vi "Execute.vi"(8 "error in (no error)":errorcluster, 10 "Abstract Consumer in":refnum<class "Abstract Consumer.lvclass">, 11 "String Request Message in":refnum<class "String Request Message.lvclass">) -> (0 "error out":errorcluster, 1 "Abstract Response out":refnum<class "Abstract Response Message.lvclass">, 2 "Abstract Consumer out":refnum<class "Abstract Consumer.lvclass">, 3 "String Request Message out":refnum<class "String Request Message.lvclass">, 4 "Stop?":bool)   [LabVIEW 2017, in "String Request Message.lvclass"]
uses:
  String Request Message.lvclass
  Consumer/Abstract Consumer/Abstract Consumer.lvclass
  Message/Abstract Response Message/Abstract Response Message.lvclass
  String Request Message.lvclass/String Request Message.ctl
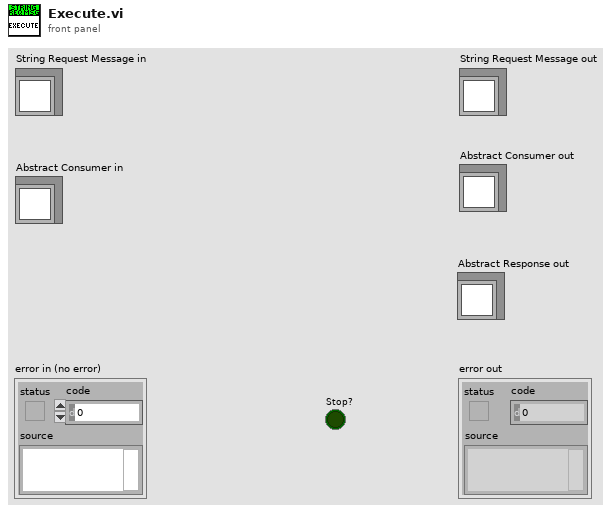
[diagram p1: front panel]
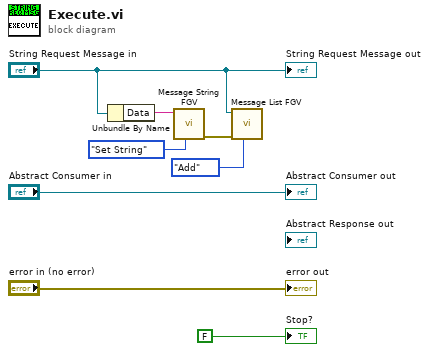
[diagram p0: block diagram]
diagram:
  n1 = Unbundle By Name("String Request Message in") -> ("Data"=w5:string)
  n2 = call "Message String FGV.vi"("Action"=enum16{"Get String", "Set String", "Reset"}."Set String", "Message String"=w5) -> ("error out"=w4:errorcluster)  [unwired: 8 in, 1 out]
  n3 = call "Message List FGV.vi"("Action (Get)"=enum16{"Get", "Add", "Reset"}."Add", "error in (no error)"=w4, "Message Object"="String Request Message in") -> ()  [unwired: 7 in, 2 out]
  "error out" <- "error in (no error)"
  "String Request Message out" <- "String Request Message in"
  "Abstract Consumer out" <- "Abstract Consumer in"
  "Stop?" <- FALSE ("Stop?")
